vi "TDTRX6-Init ActiveX.vi"(11 "error in (no error)":errorcluster) -> (4 "RPcox":refnum<k7>, 15 "error out":errorcluster)   [LabVIEW 2015]
uses:
  TDT-Globals.vi
panel:
  out "ZBUSx":refnum<k7>
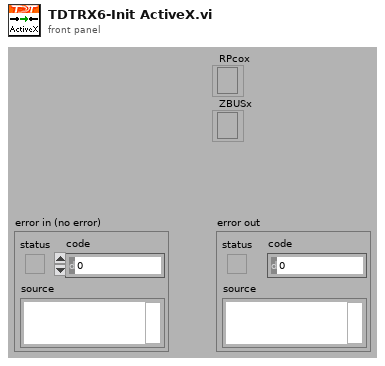
[diagram p1: front panel]
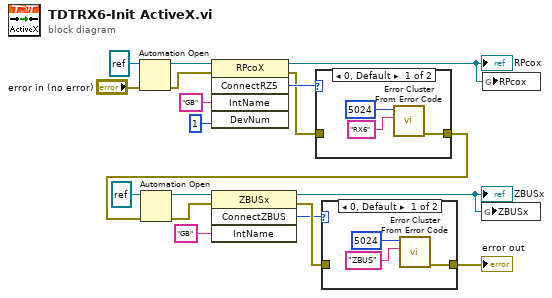
[diagram p0: block diagram]
diagram:
  n1 = Automation Open(error in (no error)="error in (no error)", Automation Refnum=refnum<k7> refnum ("RPCOXLib.RPcoX")) -> (Automation Refnum=w10:refnum<k7>, error out=w7:errorcluster)  [unwired: 2 in]
  n2 = invoke class="RPcoX" method="ConnectRZ5"(reference=w10, error in=w7, "IntName"="GB", "DevNum"=1) -> (reference out=w1:refnum<k7>, error out=w4:errorcluster, "ConnectRZ5"=w5:i32)  [unwired: 1 in, 2 out]
  "RPcox" <- w1
  n3 = case shown="0, Default" w5 {
    tunnel: w4 -> [_ w22]
    tunnel: [w19 w22] -> w3
    frame 0, Default {
      n4 = call <vilib>:"Error Cluster From Error Code.vi"("error message (\"\")"="RX6" ("error message (\"\")"), "error code (0)"=5024) -> ("error out"=w19:errorcluster)  [unwired: 7 in]
    }
    frame 1 {
    }
  }
  n5 = Automation Open(error in (no error)=w3, Automation Refnum=refnum<k7> refnum ("ZBUSXLib.ZBUSx")) -> (Automation Refnum=w16:refnum<k7>, error out=w17:errorcluster)  [unwired: 2 in]
  n6 = invoke class="ZBUSx" method="ConnectZBUS"(reference=w16, error in=w17, "IntName"="GB" ("ServerName")) -> (reference out=w2:refnum<k7>, error out=w14:errorcluster, "ConnectZBUS"=w12:i32)  [unwired: 1 in, 1 out]
  "ZBUSx" <- w2
  n7 = case shown="0, Default" w12 {
    tunnel: w14 -> [_ w26]
    tunnel: [w23 w26] -> w13
    frame 0, Default {
      n8 = call <vilib>:"Error Cluster From Error Code.vi"("error message (\"\")"="ZBUS" ("error message (\"\")"), "error code (0)"=5024) -> ("error out"=w23:errorcluster)  [unwired: 7 in]
    }
    frame 1 {
    }
  }
  "error out" <- w13
  n9 = global write "TDT-Globals.vi" "ZBUSx"(w2) -> ()
  n10 = global write "TDT-Globals.vi" "RPcox"(w1) -> ()
